vi "Measure.vi"(5 "Buffer 1":string, 6 "Buffer 2":string, 7 "Function (Current)":T1(ring), 8 "error in (no error)":errorcluster, 9 "Channel (Channel A)":T2, 10 "Node In":string, 11 "VISA resource name":refnum<visa-resource-name>) -> (0 "error out":errorcluster, 1 "Output":string, 2 "Node Out":string, 3 "VISA resource name out":refnum<visa-resource-name>, 4 "Command String":string)   [LabVIEW 2018, in "Keithley 2600 Series.lvlib"]
doc: "This VI will initiate one or more measurements.\n\n<b>Note:</b> If more than one measurement will be taken (smuX.measure.count > 1), reading buffers must be specified; otherwise, all but the last reading will be lost.\n\n<b>Functions and Attributes Used</b>\nsmuX.measure.Y()\nsmuX.measure.Y(rbuffer)\nsmuX.measure.iv(ibuffer, vbuffer)"
uses:
  Keithley 2600 Series.lvlib
  Channel.ctl
  GlobalVariables.vi
panel:
  # "(c) 2008 Keithley Instruments, Inc.  ALL RIGHTS RESERVED."
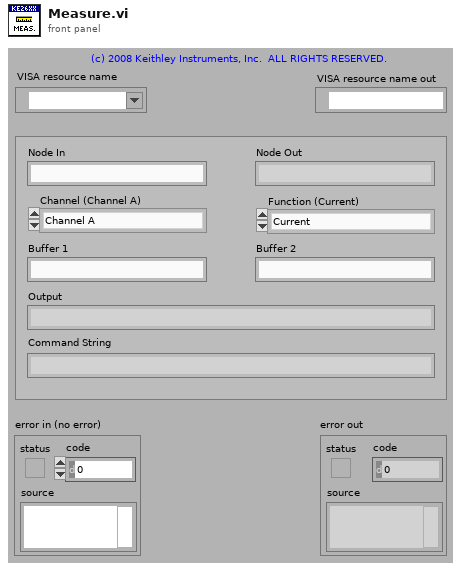
[diagram p1: front panel]
types:
  T1 = enum32{"Current", "Voltage", "IV", "Resistance", "Power"}
  T2 = typedef "Keithley 2600 Series.lvlib/Channel.ctl" = enum32{"Channel A", "Channel B"}
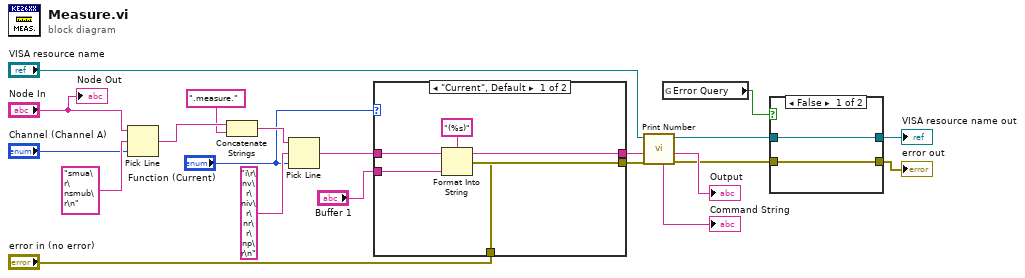
[diagram p0: block diagram]
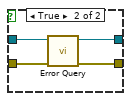
[diagram p2: hidden frame]
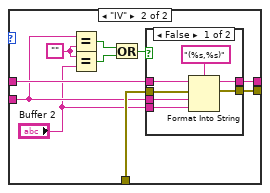
[diagram p3: hidden frame]
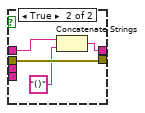
[diagram p4: hidden frame]
diagram:
  n1 = Pick Line(string ("")="Node In", multi-line string="smua\r\nsmub\r\n" ("options"), line index="Channel (Channel A)") -> (output string=w20:string)
  n2 = Concatenate Strings(w20, ".measure." ("command")) -> (w18:string)
  n3 = Pick Line(string ("")=w18, multi-line string="i\r\nv\r\niv\r\nr\r\np\r\n" ("options"), line index="Function (Current)") -> (output string=w14:string)
  n4 = case shown="\"Current\", Default" "Function (Current)" {
    tunnel: w14 -> [w26 w37]
    tunnel: "Buffer 1" -> [w22 w29]
    tunnel: [w25 w36] -> w8
    tunnel: [w24 w35] -> w9
    tunnel: "error in (no error)" -> [w23 w34]
    frame "Current", Default {
      n5 = Format Into String(format string="(%s)", initial string=w26, error in=w23, w22) -> (resulting string=w25:string, error out=w24:errorcluster)
    }
    frame "IV" {
      w30 = ""
      n6 = Equal?(x=w29, y=w30) -> (x = y?=w31:bool)
      n7 = Equal?(x=w30, y="Buffer 2") -> (x = y?=w33:bool)
      n8 = Or(x=w31, y=w33) -> (x .or. y?=w32:bool)
      n9 = case shown="False" w32 {
        tunnel: w37 -> [w43 w46]
        tunnel: [w42 w47] -> w36
        tunnel: [w41 w48] -> w35
        tunnel: w29 -> [w40 _]
        tunnel: "Buffer 2" -> [w39 _]
        tunnel: w34 -> [w38 w48]
        frame False {
          n10 = Format Into String(format string="(%s,%s)", initial string=w43, error in=w38, w40, w39) -> (resulting string=w42:string, error out=w41:errorcluster)
        }
        frame True {
          n11 = Concatenate Strings(w46, "()" ("string")) -> (w47:string)
        }
      }
    }
  }
  n12 = call "Print Number.vi"("error in (no error)"=w9, "Input"=w8, "VISA resource name"="VISA resource name") -> ("error out"=w4:errorcluster, "Output"=→"Output":string, "VISA resource name out"=w3:refnum<visa-resource-name>, "Command String"=→"Command String":string)  [unwired: 5 out]
  n13 = global read "GlobalVariables.vi" "Error Query"() -> (w5:bool)
  n14 = case shown="False" w5 {
    tunnel: w3 -> [w50 w54]
    tunnel: w4 -> [w49 w53]
    tunnel: [w50 w52] -> w2
    tunnel: [w49 w51] -> w1
    frame False {
    }
    frame True {
      n15 = call "Error Query.vi"("error in (no error)"=w53, "VISA resource name"=w54) -> ("error out"=w51:errorcluster, "VISA resource name out"=w52:refnum<visa-resource-name>)  [unwired: 8 out]
    }
  }
  "VISA resource name out" <- w2
  "error out" <- w1
  "Node Out" <- "Node In"
